vi "Write Report.vi"(8 "error in (no error)":errorcluster, 10 "Resource In":variant, 11 "Target Point in":refnum<class "Target Point.lvclass">) -> (0 "error out":errorcluster, 2 "Resource Out":variant, 3 "Target Point out":refnum<class "Target Point.lvclass">)   [LabVIEW 2014, in "Target Point.lvclass"]
uses:
  Target Point.lvclass
  <vilib>/Utility/config.llb/Config Data RefNum.ctl
  Target Point.lvclass/Target Point.ctl
  <vilib>/Utility/config.llb/Write Key (Double).vi
  <vilib>/Utility/config.llb/NI_LVConfig.lvlib
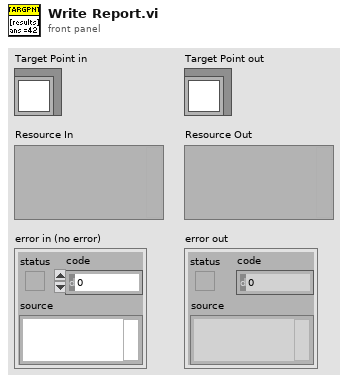
[diagram p1: front panel]
types:
  T1 = typedef "NI_LVConfig.lvlib/Config Data RefNum.ctl" = refnum<k1>
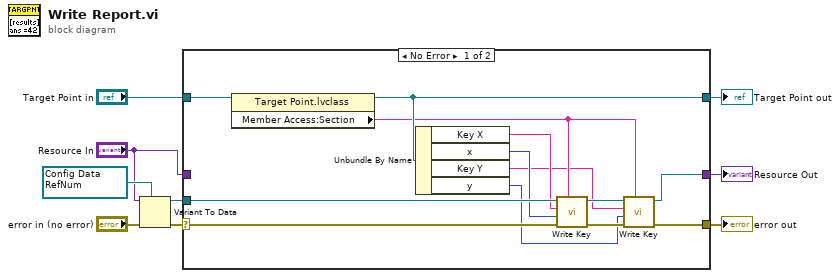
[diagram p0: block diagram]
diagram:
  w9 = T1 refnum items=["config data"] ("refnum")
  n1 = Variant To Data(error in="error in (no error)", type=w9, Variant="Resource In") -> (data=w8:T1, error out=w7:errorcluster)
  n2 = case shown="No Error" w7 {
    selector: w7 -> [w13 w24]
    tunnel: w8 -> [w22 _]
    tunnel: "Target Point in" -> [w21 w23]
    tunnel: [w20 w23] -> w3
    tunnel: [w18 w25] -> w2
    tunnel: [w17 w24] -> w1
    tunnel: "Resource In" -> [_ w25]
    frame No Error {
      n3 = property class="Target Point.lvclass"(reference=w21) -> (reference out=w20:refnum<class "Target Point.lvclass">, "Member Access:Section"=w16:string)  [unwired: 1 in, 1 out]
      n4 = Unbundle By Name(w20) -> ("Key X"=w11:string, "x"=w19:i16, "Key Y"=w10:string, "y"=w12:i16)
      n5 = call-poly <vilib>:"Write Key.vi"("section"=w16, "error in (no error)"=w13, "value"=w19, "key"=w11, "refnum"=w22) -> ("error out"=w15:errorcluster, "refnum out"=w14:T1)  [unwired: 4 in, 1 out]
      n6 = call-poly <vilib>:"Write Key.vi"("section"=w16, "error in (no error)"=w15, "value"=w12, "key"=w10, "refnum"=w14) -> ("error out"=w17:errorcluster, "refnum out"=w18:T1)  [unwired: 4 in, 1 out]
    }
    frame Error {
    }
  }
  "error out" <- w1
  "Target Point out" <- w3
  "Resource Out" <- w2
